vi "Hardware In - NI 9757-1 (O2).vi"(9 "UEGOBackPressure [bar] (1.013)":sgl=1.013, 10 "Sync":bool, 11 "FPGA Ref":T1) -> (3 "O2-1":T2)   [LabVIEW 2015, in "ECS-RT.lvlib"]
uses:
  ECS-RT.lvlib
  Typedefs/Raw Inputs/NI9757.ctl
  Typedefs/FPGA Refs/Generic FPGA Ref.ctl
  <vilib>/Utility/error.llb/Error Cluster From Error Code.vi
  <vilib>/rvi/errors/niLvFpgaAdjustHostInterfaceError.vi
  <vilib>/rvi/interface/nirviReadWriteControl/nirviReadWriteControl.xnode
  <vilib>/rvi/interface/Simulation/niFpgaSimulationCallBeginRW.vi
  ECS-Shared.lvlib
  NiFpgaLv.dll
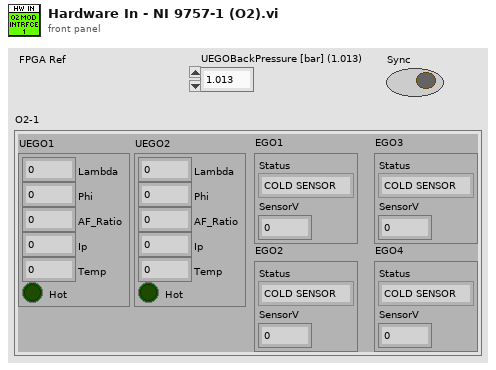
[diagram p1: front panel]
types:
  T1 = typedef "ECS-Shared.lvlib/Generic FPGA Ref.ctl" = refnum<k20>
  T2 = typedef "ECS-Shared.lvlib/NI9757.ctl" = cluster{"UEGO1":cluster{"Lambda":sgl, "Phi":sgl, "AF_Ratio":sgl, "Ip":sgl, "Temp":sgl, "Hot":bool}, "UEGO2":cluster{"Lambda":sgl, "Phi":sgl, "AF_Ratio":sgl, "Ip":sgl, "Temp":sgl, "Hot":bool}, "EGO1":cluster{"Status":enum16{"COLD SENSOR", "FOULED SENSOR", "RICH", "LEAN"}, "SensorV":sgl}, "EGO2":cluster{"Status":enum16{"COLD SENSOR", "FOULED SENSOR", "RICH", "LEAN"}, "SensorV":sgl}, "EGO3":cluster{"Status":enum16{"COLD SENSOR", "FOULED SENSOR", "RICH", "LEAN"}, "SensorV":sgl}, "EGO4":cluster{"Status":enum16{"COLD SENSOR", "FOULED SENSOR", "RICH", "LEAN"}, "SensorV":sgl}}
  T3 = cluster{"UEGO1Enable":bool, "UEGO2Enable":bool, "EGO1Enable":bool, "EGO2Enable":bool, "EGO3Enable":bool, "EGO4Enable":bool, "UEGO1Range":bool, "UEGO2Range":bool, "FilterCutoff (Hz)":dbl}
  T4 = enum32{"Diesel", "Gasoline PFI", "Stoich GDI", "Dual Fuel"}
  T5 = cluster{"UEGO1BackPressure (bar)":sgl, "UEGO2BackPressure (bar)":sgl}
  T6 = cluster{"UEGO1Diag":u8, "UEGO2Diag":u8, "UEGO1Sensor":u16, "UEGO2Sensor":u16, "UEGO1Heater":u16, "UEGO2Heater":u16, "UEGO1AmpOffset":u16, "UEGO2AmpOffset":u16, "UEGO1RIOffset":u16, "UEGO2RIOffset":u16, "UEGO1HeaterGain":u16, "UEGO2HeaterGain":u16, "Fuse":u16, "EGO1Sensor":u16, "EGO2Sensor":u16, "EGO3Sensor":u16, "EGO4Sensor":u16, "Battery":u16, "ModulePresent":bool, "UEGO1ID":u8, "UEGO2ID":u8, "LSUType":u8}
  T7 = cluster{"Stoich A/F Ratio":sgl, "IpArray (mA)":sgl[], "LambdaArray":sgl[]}
  T8 = cluster{"ModulePresent":bool, "UEGO1SensorFault":u8, "UEGO2SensorFault":u8, "UEGO1HeaterFault":u8, "UEGO2HeaterFault":u8, "UEGOFuseStatus":u8, "Battery (V)":sgl, "LSUType":u8}
  T9 = cluster{"UEGO1Lambda":sgl, "UEGO1Phi":sgl, "UEGO1AFRatio":sgl, "UEGO1Ip (mA)":sgl, "UEGO2Lambda":sgl, "UEGO2Phi":sgl, "UEGO2AFRatio":sgl, "UEGO2Ip (mA)":sgl}
  T10 = cluster{"EGO1Status":u8, "EGO2Status":u8, "EGO3Status":u8, "EGO4Status":u8, "EGO1Sensor (V)":sgl, "EGO2Sensor (V)":sgl, "EGO3Sensor (V)":sgl, "EGO4Sensor (V)":sgl}
  T11 = cluster{"UEGO1Heater (V)":sgl, "UEGO2Heater (V)":sgl}
  T12 = cluster{"UEGO1Temp (C)":sgl, "UEGO2Temp (C)":sgl, "UEGO1Hot":bool, "UEGO2Hot":bool}
  T13 = cluster{"ModuleEnable":bool, "WatchdogIn":bool, "UEGO1Hot":bool, "UEGO2Hot":bool, "Cal1Request":bool, "Cal2Request":bool, "UEGOHeaterPeriod":u16, "UEGO1HeaterPulseWidth":u16, "UEGO2HeaterPulseWidth":u16, "UEGO1Range":bool, "UEGO2Range":bool, "LSUType (F=4.9,T=4.2)":bool}
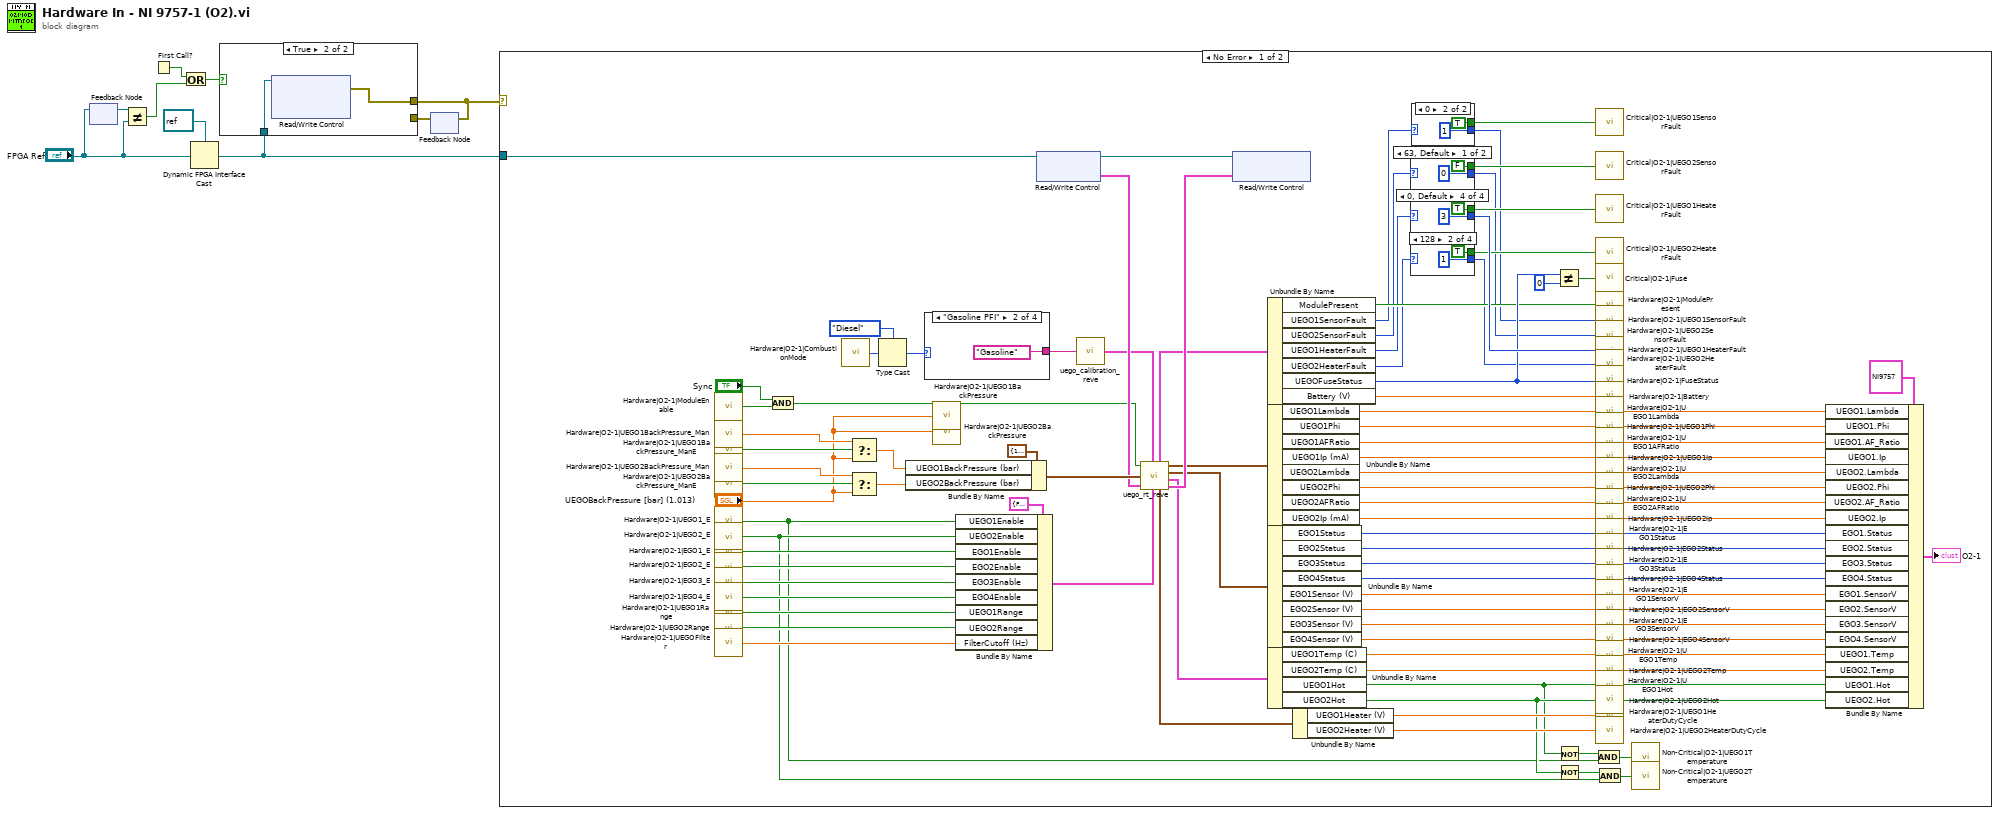
[diagram p0: block diagram]
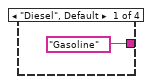
[diagram p3: hidden frame]
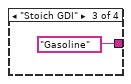
[diagram p4: hidden frame]
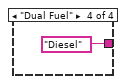
[diagram p5: hidden frame]
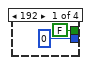
[diagram p6: hidden frame]
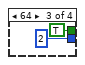
[diagram p7: hidden frame]
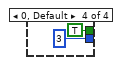
[diagram p8: hidden frame]
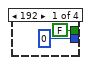
[diagram p9: hidden frame]
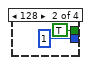
[diagram p10: hidden frame]
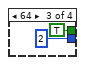
[diagram p11: hidden frame]
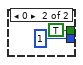
[diagram p12: hidden frame]
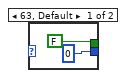
[diagram p13: hidden frame]
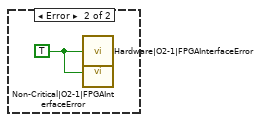
[diagram p14: hidden frame]
diagram:
  n1 = feedback #1() -> (w8:T1)  [unwired: 1 in]
  n2 = feedback-in #1("FPGA Ref") -> ()
  n3 = Not Equal?(x=w8, y="FPGA Ref") -> (x != y?=w9:bool)
  n4 = First Call?() -> (First Call?: T/F=w7:bool)
  n5 = Or(x=w7, y=w9) -> (x .or. y?=w6:bool)
  n6 = Dynamic FPGA Interface Cast(Session In=refnum<k20> refnum ("FPGA VI Reference Out"), Type="FPGA Ref") -> (Session Out=w1:refnum<k20>)
  n7 = feedback #2() -> (w5:errorcluster)  [unwired: 1 in]
  n8 = case shown="True" w6 {
    tunnel: [w10 w12] -> w4
    tunnel: w5 -> [w10 _]
    tunnel: w1 -> [_ w11]
    frame False {
    }
    frame True {
      n9 = xnode "Read/Write Control"("FPGA VI Reference In"=w11) -> ("error out"=w12:errorcluster)  [unwired: 2 in, 2 out]
    }
  }
  n10 = feedback-in #2(w4) -> ()
  n11 = case shown="No Error" w4 {
    tunnel: w1 -> [w41 _]
    frame No Error {
      n12 = call "Hardware|O2-1|ModuleEnable"() -> ("Value"=w15:bool)
      n13 = call "Hardware|O2-1|UEGO1BackPressure_Man"() -> ("Value"=w83:sgl)
      n14 = call "Hardware|O2-1|UEGO1BackPressure_ManE"() -> ("Value"=w80:bool)
      n15 = call "Hardware|O2-1|UEGO2BackPressure_Man"() -> ("Value"=w82:sgl)
      n16 = call "Hardware|O2-1|UEGO2BackPressure_ManE"() -> ("Value"=w81:bool)
      n17 = call "Hardware|O2-1|UEGO1_E"() -> ("Value"=w16:bool)
      n18 = call "Hardware|O2-1|UEGO2_E"() -> ("Value"=w17:bool)
      n19 = call "Hardware|O2-1|EGO1_E"() -> ("Value"=w74:bool)
      n20 = call "Hardware|O2-1|EGO2_E"() -> ("Value"=w75:bool)
      n21 = call "Hardware|O2-1|EGO3_E"() -> ("Value"=w76:bool)
      n22 = call "Hardware|O2-1|EGO4_E"() -> ("Value"=w77:bool)
      n23 = call "Hardware|O2-1|UEGO1Range"() -> ("Value"=w20:bool)
      n24 = call "Hardware|O2-1|UEGO2Range"() -> ("Value"=w22:bool)
      n25 = call "Hardware|O2-1|UEGOFilter"() -> ("Value"=w21:sgl)
      n26 = And(x="Sync", y=w15) -> (x .and. y?=w14:bool)
      n27 = call "Hardware|O2-1|CombustionMode"() -> ("Value"=w43:u32)
      n28 = Select(t=w83, s=w80, f="UEGOBackPressure [bar] (1.013)") -> (s? t:f=w79:sgl)
      n29 = Select(t=w82, s=w81, f="UEGOBackPressure [bar] (1.013)") -> (s? t:f=w78:sgl)
      n30 = Type Cast(type=T4."Diesel" ("CombustionMode"), x=w43) -> (*(type *) &x=w42:T4)
      n31 = Bundle By Name(cluster=T5 {"UEGO1BackPressure (bar)"=1.013, "UEGO2BackPressure (bar)"=1.013} ("UEGO Back Pressure (bar)"), "UEGO1BackPressure (bar)"=w79, "UEGO2BackPressure (bar)"=w78) -> (w67:T5)
      n32 = case shown="\"Gasoline PFI\"" w42 {
        tunnel: ["Gasoline" ("Fuel Selection UEGO") "Gasoline" ("Fuel Selection UEGO") "Gasoline" ("Fuel Selection UEGO") "Diesel" ("Fuel Selection UEGO")] -> w56
        frame "Diesel", Default {
        }
        frame "Gasoline PFI" {
        }
        frame "Stoich GDI" {
        }
        frame "Dual Fuel" {
        }
      }
      n33 = call "Hardware|O2-1|UEGO1BackPressure"("Value"="UEGOBackPressure [bar] (1.013)") -> ()
      n34 = call "Hardware|O2-1|UEGO2BackPressure"("Value"="UEGOBackPressure [bar] (1.013)") -> ()
      n35 = Bundle By Name(cluster=T3 {"UEGO1Enable"=FALSE, "UEGO2Enable"=FALSE, "EGO1Enable"=FALSE, "EGO2Enable"=FALSE, "EGO3Enable"=FALSE, "EGO4Enable"=FALSE, "UEGO1Range"=FALSE, "UEGO2Range"=FALSE, "FilterCutoff (Hz)"=10.0} ("SensorControl"), "UEGO1Enable"=w16, "UEGO2Enable"=w17, "EGO1Enable"=w74, "EGO2Enable"=w75, "EGO3Enable"=w76, "EGO4Enable"=w77, "UEGO1Range"=w20, "UEGO2Range"=w22, "FilterCutoff (Hz)"=w21) -> (w23:T3)
      n36 = xnode "Read/Write Control"("FPGA VI Reference In"=w41) -> ("FPGA VI Reference Out"=w60:refnum<k20>, "O2-1.Data"=w59:T6)  [unwired: 1 in, 1 out]
      n37 = call <vilib>:"uego_calibration_reve.vi"("Fuel Selection"=w56) -> ("UEGOCalibration"=w57:T7)
      n38 = call <vilib>:"uego_rt_reve.vi"("UEGOModuleEnable"=w14, "UEGOCalibration"=w57, "UEGO Back Pressure (bar)"=w67, "UEGOData (From FPGA)"=w59, "SensorControl"=w23) -> ("UEGO Diagnostics"=w62:T8, "UEGO Sensor Results"=w61:T9, "EGO Sensor Results"=w63:T10, "UEGO Heater (V)"=w65:T11, "UEGO Temperature (C)"=w64:T12, "UEGOControl (To FPGA)"=w94:T13)
      n39 = xnode "Read/Write Control"("FPGA VI Reference In"=w60, "O2-1.Control"=w94) -> ()  [unwired: 1 in, 2 out]
      n40 = Unbundle By Name(w62) -> ("ModulePresent"=w87:bool, "UEGO1SensorFault"=w53:u8, "UEGO2SensorFault"=w69:u8, "UEGO1HeaterFault"=w71:u8, "UEGO2HeaterFault"=w73:u8, "UEGOFuseStatus"=w90:u8, "Battery (V)"=w68:sgl)
      n41 = Unbundle By Name(w61) -> ("UEGO1Lambda"=w19:sgl, "UEGO1Phi"=w52:sgl, "UEGO1AFRatio"=w51:sgl, "UEGO1Ip (mA)"=w50:sgl, "UEGO2Lambda"=w18:sgl, "UEGO2Phi"=w48:sgl, "UEGO2AFRatio"=w47:sgl, "UEGO2Ip (mA)"=w46:sgl)
      n42 = Unbundle By Name(w63) -> ("EGO1Status"=w32:u8, "EGO2Status"=w31:u8, "EGO3Status"=w30:u8, "EGO4Status"=w29:u8, "EGO1Sensor (V)"=w28:sgl, "EGO2Sensor (V)"=w27:sgl, "EGO3Sensor (V)"=w26:sgl, "EGO4Sensor (V)"=w25:sgl)
      n43 = Unbundle By Name(w64) -> ("UEGO1Temp (C)"=w33:sgl, "UEGO2Temp (C)"=w34:sgl, "UEGO1Hot"=w35:bool, "UEGO2Hot"=w36:bool)
      n44 = Unbundle By Name(w65) -> ("UEGO1Heater (V)"=w92:sgl, "UEGO2Heater (V)"=w93:sgl)
      n45 = case shown="63, Default" w69 {
        tunnel: [0 1] -> w70
        tunnel: [FALSE TRUE] -> w86
        frame 63, Default {
        }
        frame 0 {
        }
      }
      n46 = case shown="0, Default" w71 {
        tunnel: [0 1 2 3] -> w91
        tunnel: [FALSE TRUE TRUE TRUE] -> w85
        frame 192 {
        }
        frame 128 {
        }
        frame 64 {
        }
        frame 0, Default {
        }
      }
      n47 = case shown="128" w73 {
        tunnel: [0 1 2 3] -> w72
        tunnel: [FALSE TRUE TRUE TRUE] -> w84
        frame 192 {
        }
        frame 128 {
        }
        frame 64 {
        }
        frame 0, Default {
        }
      }
      n48 = case shown="0" w53 {
        tunnel: [FALSE TRUE] -> w55
        tunnel: [0 1] -> w54
        frame 63, Default {
        }
        frame 0 {
        }
      }
      n49 = Not Equal?(x=w90, y=0) -> (x != y?=w89:bool)
      n50 = Not(x=w35) -> (.not. x?=w38:bool)
      n51 = Not(x=w36) -> (.not. x?=w37:bool)
      n52 = And(x=w38, y=w16) -> (x .and. y?=w39:bool)
      n53 = call "Critical|O2-1|UEGO1SensorFault"("Fault"=w55) -> ()  [unwired: 2 in]
      n54 = call "Critical|O2-1|UEGO2SensorFault"("Fault"=w86) -> ()  [unwired: 2 in]
      n55 = call "Critical|O2-1|UEGO1HeaterFault"("Fault"=w85) -> ()  [unwired: 2 in]
      n56 = call "Critical|O2-1|UEGO2HeaterFault"("Fault"=w84) -> ()  [unwired: 2 in]
      n57 = call "Critical|O2-1|Fuse"("Fault"=w89) -> ()  [unwired: 2 in]
      n58 = call "Hardware|O2-1|ModulePresent"("Value"=w87) -> ()
      n59 = call "Hardware|O2-1|UEGO1SensorFault"("Value"=w54) -> ()
      n60 = call "Hardware|O2-1|UEGO2SensorFault"("Value"=w70) -> ()
      n61 = call "Hardware|O2-1|UEGO1HeaterFault"("Value"=w91) -> ()
      n62 = call "Hardware|O2-1|UEGO2HeaterFault"("Value"=w72) -> ()
      n63 = call "Hardware|O2-1|FuseStatus"("Value"=w90) -> ()
      n64 = call "Hardware|O2-1|Battery"("Value"=w68) -> ()
      n65 = call "Hardware|O2-1|UEGO1Lambda"("Value"=w19) -> ()
      n66 = call "Hardware|O2-1|UEGO1Phi"("Value"=w52) -> ()
      n67 = call "Hardware|O2-1|UEGO1AFRatio"("Value"=w51) -> ()
      n68 = call "Hardware|O2-1|UEGO1Ip"("Value"=w50) -> ()
      n69 = call "Hardware|O2-1|UEGO2Lambda"("Value"=w18) -> ()
      n70 = call "Hardware|O2-1|UEGO2Phi"("Value"=w48) -> ()
      n71 = call "Hardware|O2-1|UEGO2AFRatio"("Value"=w47) -> ()
      n72 = call "Hardware|O2-1|UEGO2Ip"("Value"=w46) -> ()
      n73 = call "Hardware|O2-1|EGO1Status"("Value"=w32) -> ()
      n74 = call "Hardware|O2-1|EGO2Status"("Value"=w31) -> ()
      n75 = call "Hardware|O2-1|EGO3Status"("Value"=w30) -> ()
      n76 = call "Hardware|O2-1|EGO4Status"("Value"=w29) -> ()
      n77 = call "Hardware|O2-1|EGO1SensorV"("Value"=w28) -> ()
      n78 = call "Hardware|O2-1|EGO2SensorV"("Value"=w27) -> ()
      n79 = call "Hardware|O2-1|EGO3SensorV"("Value"=w26) -> ()
      n80 = call "Hardware|O2-1|EGO4SensorV"("Value"=w25) -> ()
      n81 = call "Hardware|O2-1|UEGO1Temp"("Value"=w33) -> ()
      n82 = call "Hardware|O2-1|UEGO2Temp"("Value"=w34) -> ()
      n83 = call "Hardware|O2-1|UEGO1Hot"("Value"=w35) -> ()
      n84 = call "Hardware|O2-1|UEGO2Hot"("Value"=w36) -> ()
      n85 = call "Hardware|O2-1|UEGO1HeaterDutyCycle"("Value"=w92) -> ()
      n86 = call "Hardware|O2-1|UEGO2HeaterDutyCycle"("Value"=w93) -> ()
      n87 = And(x=w37, y=w17) -> (x .and. y?=w40:bool)
      n88 = call "Non-Critical|O2-1|UEGO1Temperature"("Fault"=w39) -> ()  [unwired: 2 in]
      n89 = call "Non-Critical|O2-1|UEGO2Temperature"("Fault"=w40) -> ()  [unwired: 2 in]
      n90 = Bundle By Name(cluster=T2 {"UEGO1"={"Lambda"=0.0, "Phi"=0.0, "AF_Ratio"=0.0, "Ip"=0.0, "Temp"=0.0, "Hot"=FALSE}, "UEGO2"={"Lambda"=0.0, "Phi"=0.0, "AF_Ratio"=0.0, "Ip"=0.0, "Temp"=0.0, "Hot"=FALSE}, "EGO1"={"Status"=enum."COLD SENSOR", "SensorV"=0.0}, "EGO2"={"Status"=enum."COLD SENSOR", "SensorV"=0.0}, "EGO3"={"Status"=enum."COLD SENSOR", "SensorV"=0.0}, "EGO4"={"Status"=enum."COLD SENSOR", "SensorV"=0.0}} ("O2"), "UEGO1.Lambda"=w19, "UEGO1.Phi"=w52, "UEGO1.AF_Ratio"=w51, "UEGO1.Ip"=w50, "UEGO2.Lambda"=w18, "UEGO2.Phi"=w48, "UEGO2.AF_Ratio"=w47, "UEGO2.Ip"=w46, "EGO1.Status"=w32, "EGO2.Status"=w31, "EGO3.Status"=w30, "EGO4.Status"=w29, "EGO1.SensorV"=w28, "EGO2.SensorV"=w27, "EGO3.SensorV"=w26, "EGO4.SensorV"=w25, "UEGO1.Temp"=w33, "UEGO2.Temp"=w34, "UEGO1.Hot"=w35, "UEGO2.Hot"=w36) -> (→"O2-1":T2)
    }
    frame Error {
      w123 = TRUE ("Value")
      n91 = call "Hardware|O2-1|FPGAInterfaceError"("Value"=w123) -> ()
      n92 = call "Non-Critical|O2-1|FPGAInterfaceError"("Fault"=w123) -> ()  [unwired: 2 in]
    }
  }
